vi "init.vi"(8 "error in (no error)":errorcluster, 9 "Samples To Average":i32, 10 "Vref Channel":refnum<k21>, 11 "ConvertROTRawToEngStrategy in":refnum<class "ConvertROTRawToEngStrategy.lvclass">) -> (0 "error out":errorcluster, 3 "ConvertROTRawToEngStrategy out":refnum<class "ConvertROTRawToEngStrategy.lvclass">)   [LabVIEW 2015, in "ConvertROTRawToEngStrategy.lvclass"]
uses:
  ConvertROTRawToEngStrategy.lvclass
  ConvertROTRawToEngStrategy.lvclass/ConvertROTRawToEngStrategy.ctl
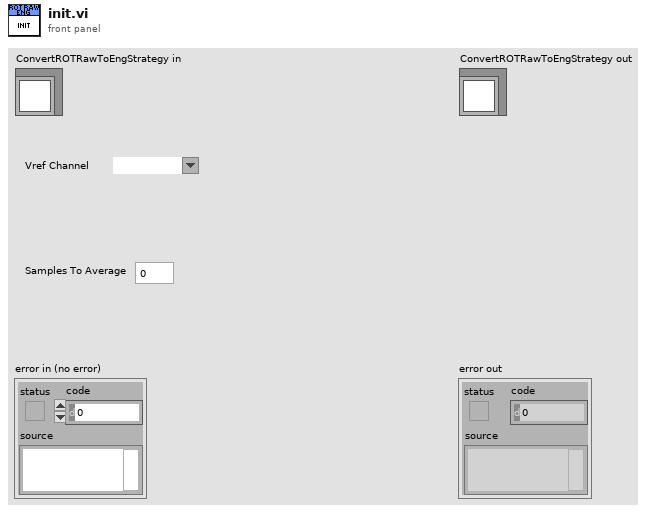
[diagram p1: front panel]
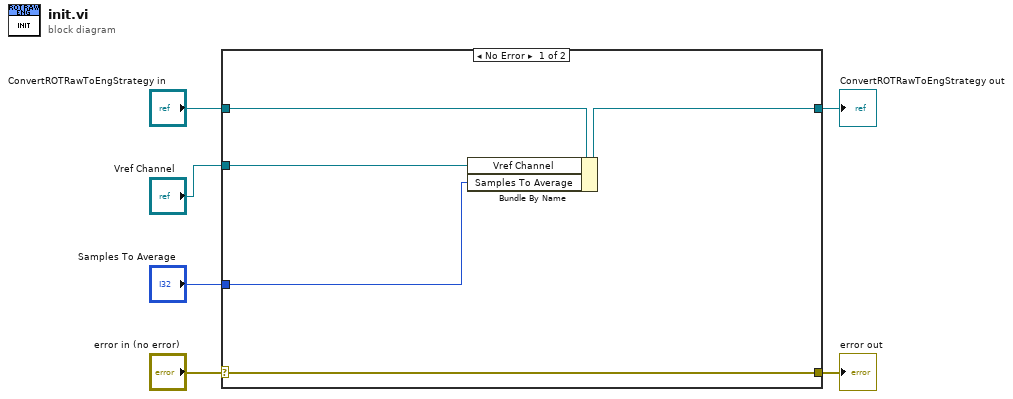
[diagram p0: block diagram]
diagram:
  n1 = case shown="No Error" "error in (no error)" {
    selector: "error in (no error)" -> [w11 w13]
    tunnel: [w11 w13] -> w5
    tunnel: [w7 w12] -> w3
    tunnel: "ConvertROTRawToEngStrategy in" -> [w8 w12]
    tunnel: "Vref Channel" -> [w10 _]
    tunnel: "Samples To Average" -> [w9 _]
    frame No Error {
      n2 = Bundle By Name(cluster=w8, "Vref Channel"=w10, "Samples To Average"=w9) -> (w7:refnum<class "ConvertROTRawToEngStrategy.lvclass">)
    }
    frame Error {
    }
  }
  "error out" <- w5
  "ConvertROTRawToEngStrategy out" <- w3
